vi "MDO-Monitor desktop1.vi"() -> ()   [LabVIEW 2012]
uses:
  SubVI/Controls/main_states.ctl
  SubVI/Controls/Globol_Data_Cluster.ctl
  SubVI/Controls/options.ctl
  SubVI/Controls/main_tab.ctl
  SubVI/Controls/process condition.ctl
  SubVI/Controls/MBA_data.ctl
  <vilib>/Utility/error.llb/DialogType.ctl
  <vilib>/Utility/file.llb/Write To Spreadsheet File (string).vi
  <vilib>/Analysis/baseanly.llb/Mean (DBL).vi
  <vilib>/Analysis/NI_AALBase.lvlib
panel:
  in  "Reset_data":bool
  in  "Пауза":bool
  in  "Принудительный запуск":bool
  in  "Отложенный запуск":bool
  in  "СТОП":bool
  out "ДАННЫЕ СОХРАНЕНЫ":string="ДАННЫЕ СОХРАНЕНЫ"
  in  "Save_data":bool
  in  "ПРИМЕЧАНИЕ":bool
  in  "ТОК ТОЧНО":u8(slide)=5 max=10 step=1 scale=0.0..10.0
  in  "ТОК ГРУБО":u8(slide)=1 max=2 step=1 scale=0.0..2.0
  in  "ПРЕДЕЛЫ ПО НАПРЯЖ":bool=TRUE
  in  "StopUgasanie":bool caption="Остановка по угасанию"
  out "ТАЙМЕР Текущий":string
  out "УГАСАНИЕ":string="УГАСАНИЕ"
  out "ДР":string="Д Р"
  out "ИР":string="И Р"
  out "ГАЛЬВ.ЛЮМ.":string="ГАЛЬВ"
  out "МДР":string="МДР"
  out "СБОР":string="СБОР"
  out "Bounds:Area Width":u32
  in  "СТОП - КАДР":bool
  in  "Graph Tab":T1(tab)
  out "Mixed Signal Graph":T2(graph)
  out "FormCharts":T3(graph) caption="Формовочные кривые"
  out "Process Electrical Parameters":string[][](table)
  out "Bath type":string caption="Ванна"
  out "Electrolyte temperature":dbl(slide) caption="Температура электролита" scale=0.0..60.0
  out "Cooler flow":dbl(knob) caption="Давление воды в системе охлаждения" scale=0.0..3.5 scale format="%#_2g"
  out "Bubbling flow":bool caption="Расход газа в барботере"
  out "Ventilation flow":bool caption="Расход газа в вытяжке"
  out "Application Directory":path
  out "Max_voltage":dbl
  out "states_history":string
  out "current_state":T4
  # "ПАНЕЛЬ ЗАПУСКА"
  # "ПУСК СЛЕДЯЩИЙ"
  # "ПУСК ПРИНУДИТ"
  # "ПАУЗА"
  # "СТОП"
  # "ПАНЕЛЬ ИНДИКАЦИИ"
  # "ПАНЕЛЬ УПРАВЛЕНИЯ"
  # "ПРЕДЕЛЫ\nПО НАПРЯЖ"
  # "800 /200"
  # "1000 / 250"
  # "СОБРАННЕ\nДАННЫЕ"
  # "ПРЕДЕЛЫ\nПО ТОКУ"
  # "ГРУБО"
  # "ТОЧНО"
  # "о"
  # "С"
  # "атм"
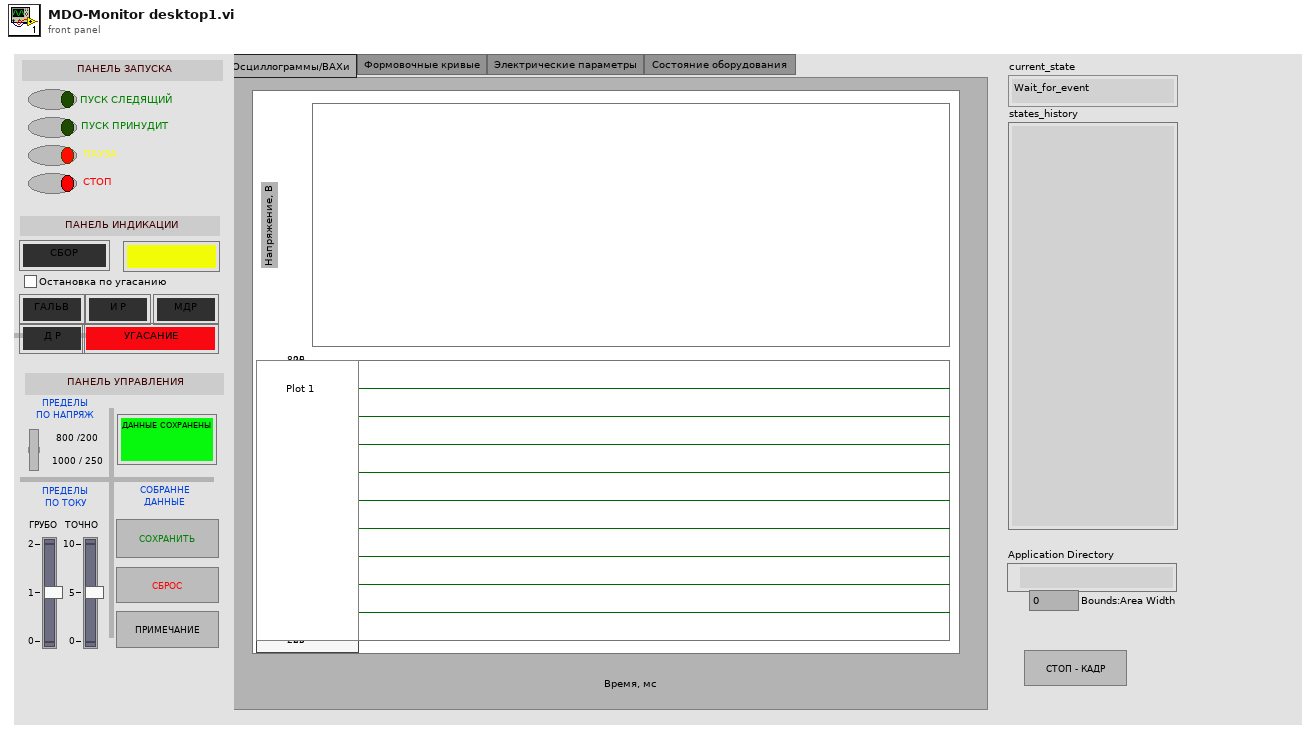
[diagram p1: front panel]
types:
  T1 = enum32{"Осциллограммы/ВАХи", "Формовочные кривые", "Электрические параметры", "Состояние оборудования "}
  T2 = cluster{"Voltege waveform":waveform(dbl), "Current waveform":waveform(dbl)}
  T3 = cluster{"Anod_amp":dbl, "Anod_rms":dbl, "Anod_mean":dbl, "Katod_amp":dbl, "Katod_rms":dbl, "Katod_mean":dbl, "Anod_amp":dbl, "Anod_rms":dbl, "Anod_mean":dbl, "Katod_amp":dbl, "Katod_rms":dbl, "Katod_mean":dbl}
  T4 = typedef "main_states.ctl" = enum16{"Wait_for_event", "Initialize", "Save_ini", "Save_data", "Streaming_config", "Streaming_open", "Streaming_monitor", "Streaming_stop", "Vizualyze", "Form_data_fetch", "Process_analyze", "Start_data_loging", "Pause_data_loging", "Stop_data_loging", "Reset_data_colection", "Error_handler", "Stop", "Settings_dialog"}
  T5 = typedef "Globol_Data_Cluster.ctl" = cluster{"Streaming_enable":bool, "Options":T6, "Ini_file_path":path, "Global_errors":errorcluster, "Main Tab":T7, "Process conditions":T8, "App_directory_path":path, "Data_write_enable":bool, "Process_time":u32, "startup_time":u32, "Streaming Refnum":refnum<vi>, "Note Refnum":refnum<vi>, "Note":string, "Modbus spy Refnum":refnum<vi>, "MBA data":T9, "shutdown?":bool, "Oscil_path":path, " Data log path":path, "Voltege waveform":waveform(dbl), "Current waveform":waveform(dbl)}
  T6 = typedef "options.ctl" = cluster{"Form_data_log_period":i32, "startup_threshold":dbl, "Coeff_U":dbl, "Offset_U":dbl, "Coeff_I":dbl, "Offset_I":dbl, "Save_data_path":path, "ADC_frequency":dbl, "VISA resource name":refnum<visa-resource-name>}
  T7 = typedef "main_tab.ctl" = enum32{"Выбор", "Описание эксперимента", "Монитор", "Визуализатор", "Принтер", "Настройщик"}
  T8 = typedef "process condition.ctl" = cluster{"Data":string, "Time":string, "Subject":string, "Research target":string, "Material":string, "Electrolyte composition":string[][], "MDO mode":string, "Bath volume":string, "Process duration":i32}
  T9 = typedef "MBA_data.ctl" = cluster{"MBA_ch 1":dbl, "MBA_ch 2":dbl, "MBA_ch 3":dbl, "MBA_ch 4":dbl, "MBA_ch 5":dbl, "MBA_ch 6":dbl, "MBA_ch 7":dbl, "MBA_ch 8":dbl}
  T10 = cluster{"Anod_amp":dbl, "Anod_rms":dbl, "Anod_mean":dbl, "Katod_amp":dbl, "Katod_rms":dbl, "Katod_mean":dbl, "Anod_amp":dbl, "Anod_rms":dbl, "Anod_mean":dbl, "Katod_amp":dbl, "Katod_rms":dbl, "Katod_mean":dbl}[]
  T11 = enum16{"open", "replace", "create", "open or create", "replace or create", "replace or create with confirmation"}
  T12 = enum8{"Enabled", "Disabled", "Disabled and Grayed Out"}
  T13 = enum32{"invalid app kind", "Development System", "Run Time System", "Student Edition", "Embedded LabVIEW", "Evaluation", "Custom"}
  T14 = cluster{"Katod_amp":dbl, "Katod_rms":dbl, "Katod_mean":dbl}
  T15 = cluster{"Katod_amp":string, "Katod_rms":string, "Katod_mean":string}
  T16 = cluster{"Anod_amp":dbl, "Anod_rms":dbl, "Anod_mean":dbl}
  T17 = cluster{"Anod_amp":string, "Anod_rms":string, "Anod_mean":string}
  T18 = typedef "DialogType.ctl" = u16
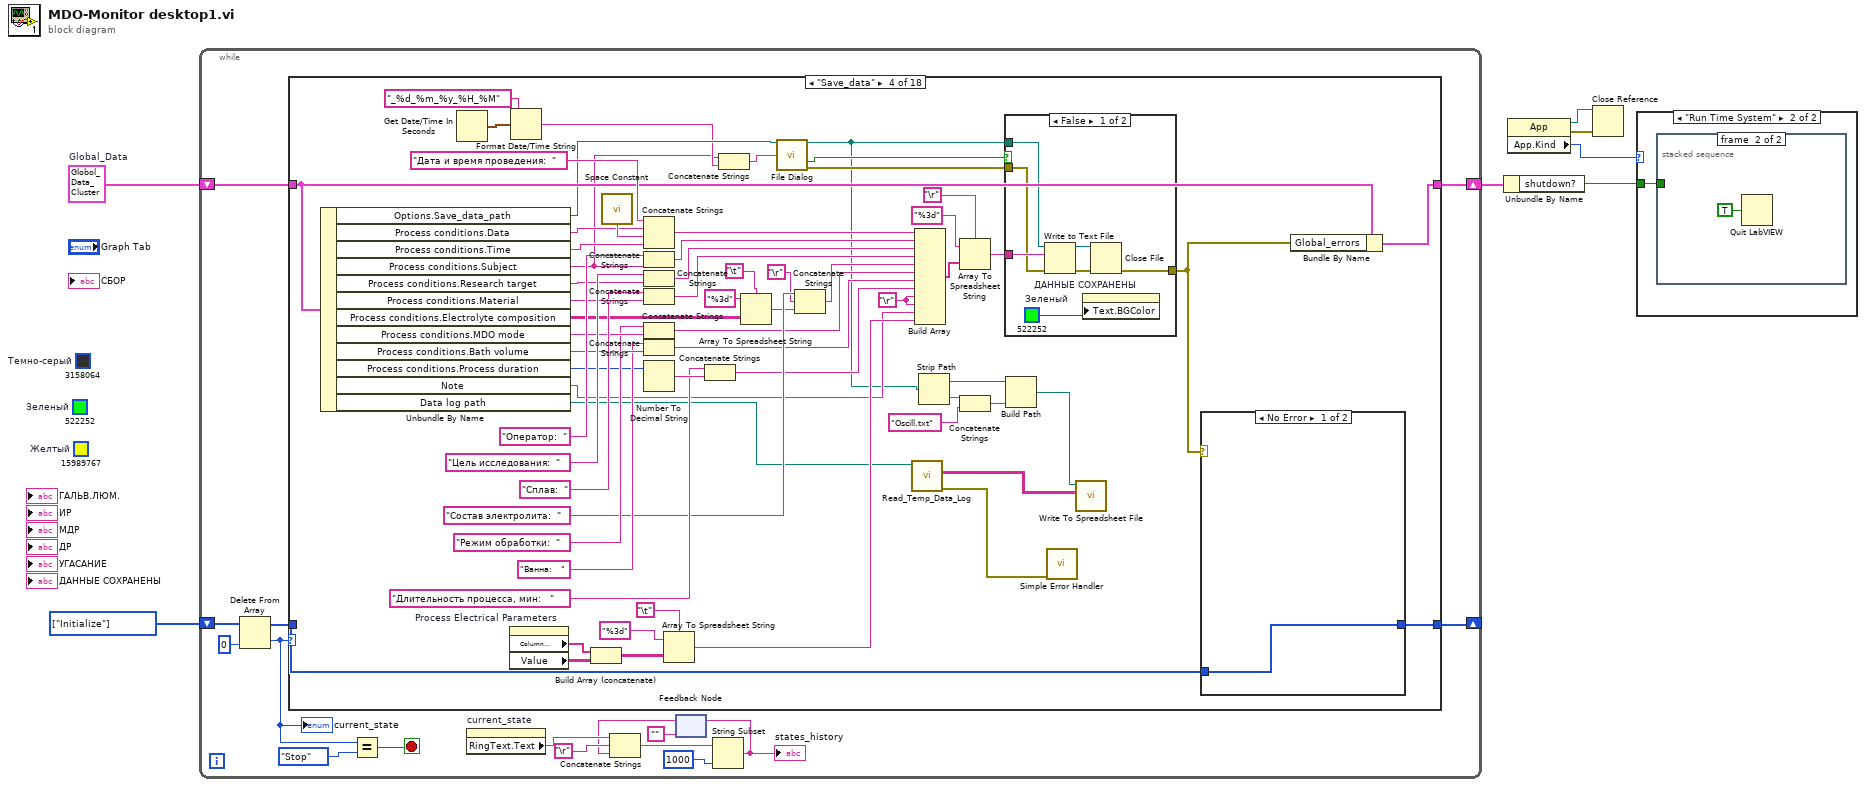
[diagram p0: block diagram]
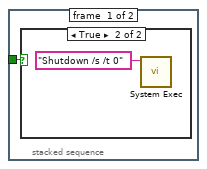
[diagram p3: hidden frame]
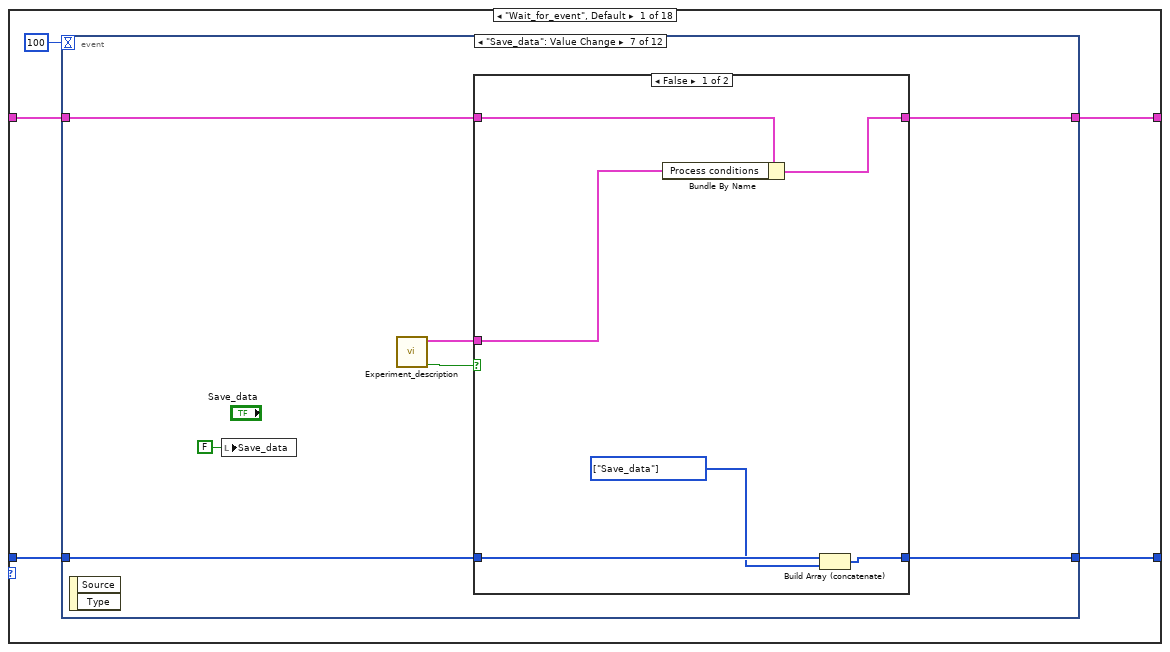
[diagram p5: hidden frame]
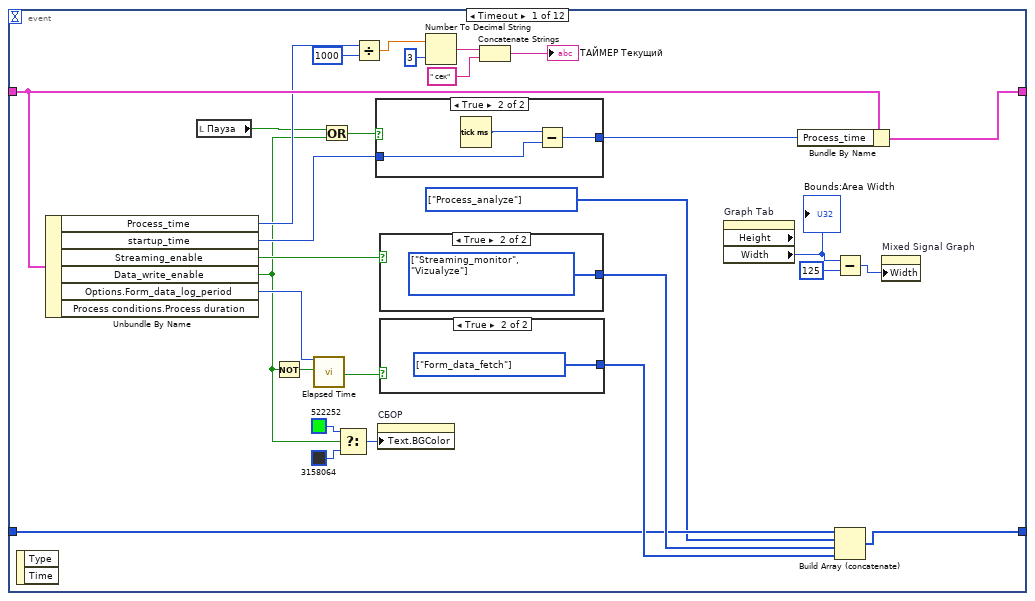
[diagram p6: hidden frame]
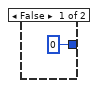
[diagram p7: hidden frame]
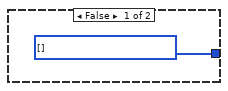
[diagram p8: hidden frame]
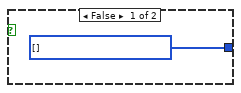
[diagram p9: hidden frame]
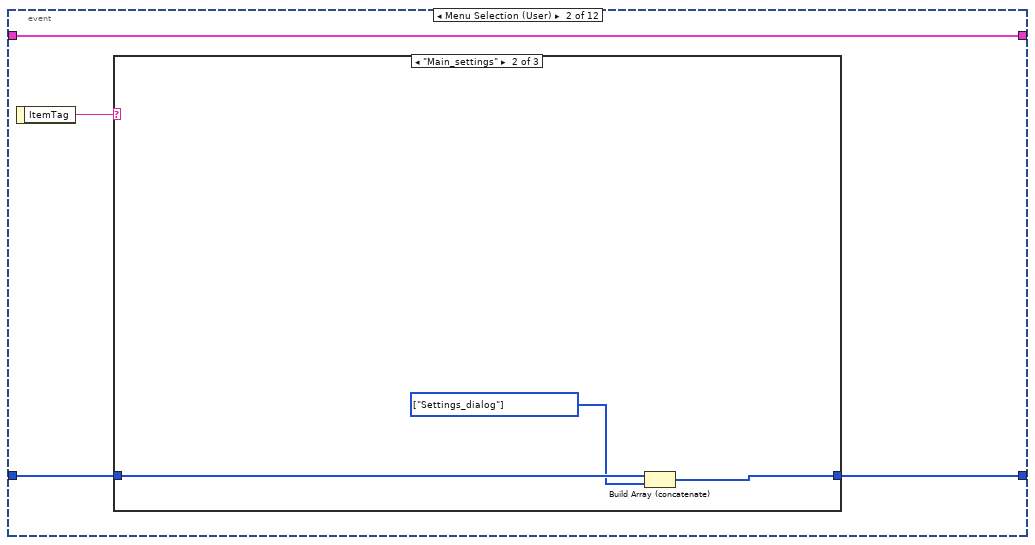
[diagram p10: hidden frame]
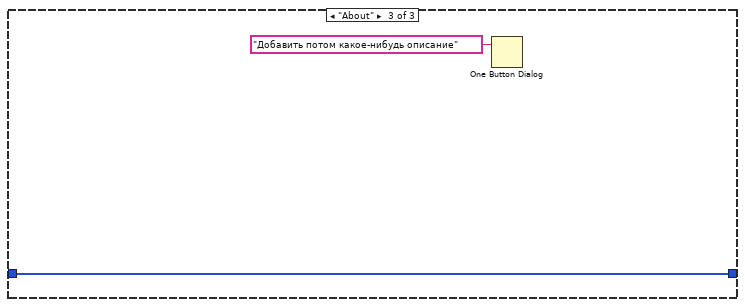
[diagram p12: hidden frame]
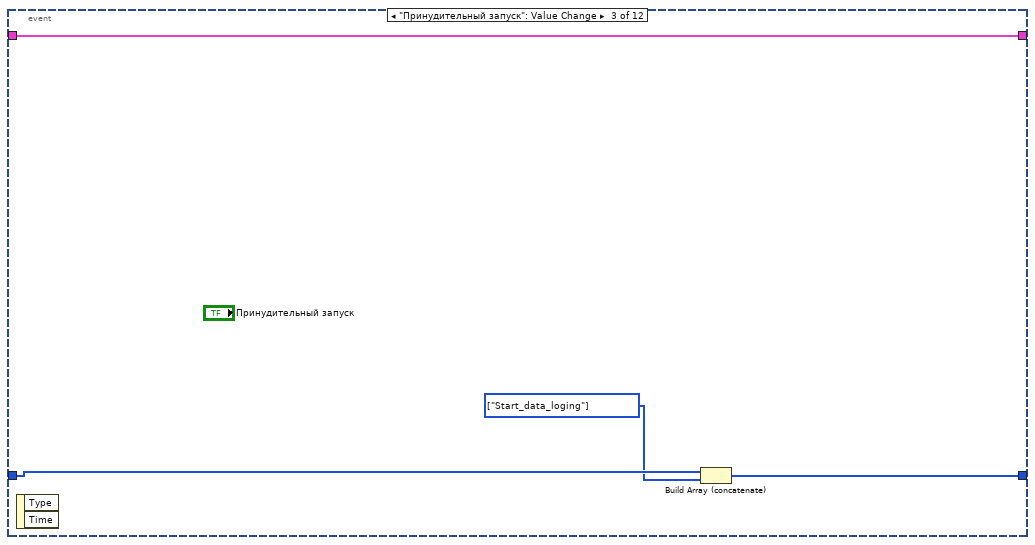
[diagram p13: hidden frame]
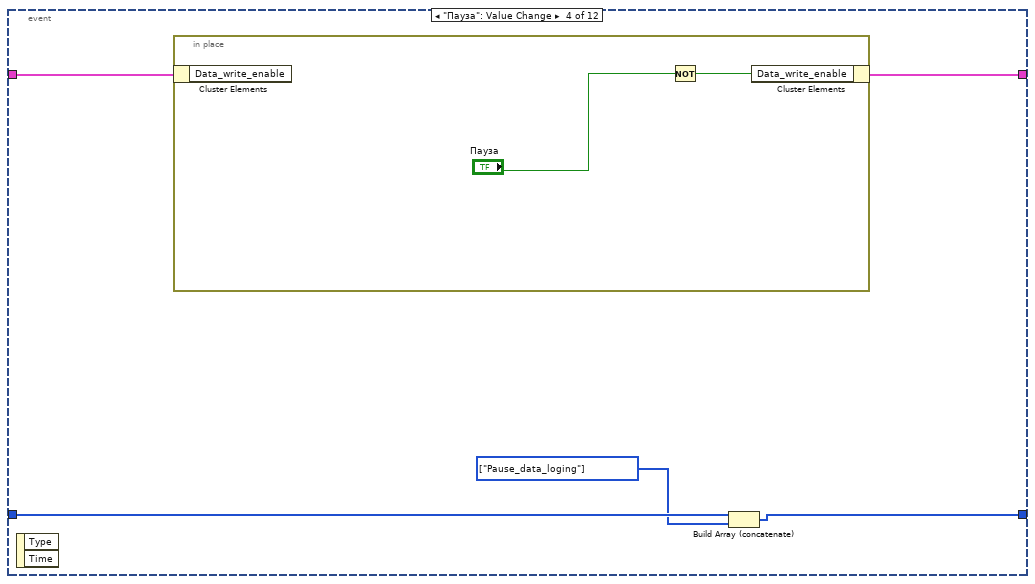
[diagram p14: hidden frame]
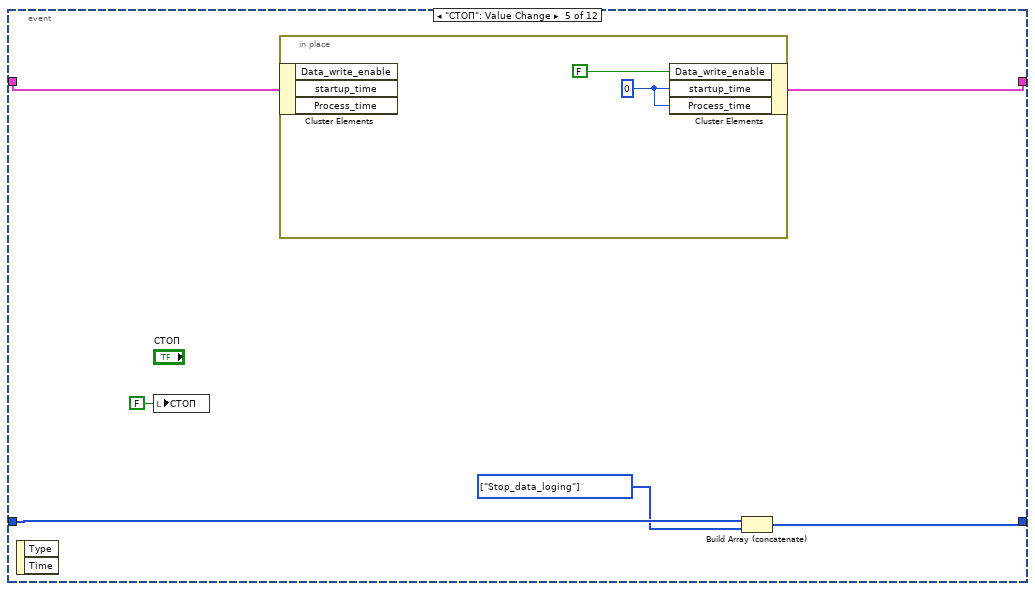
[diagram p15: hidden frame]
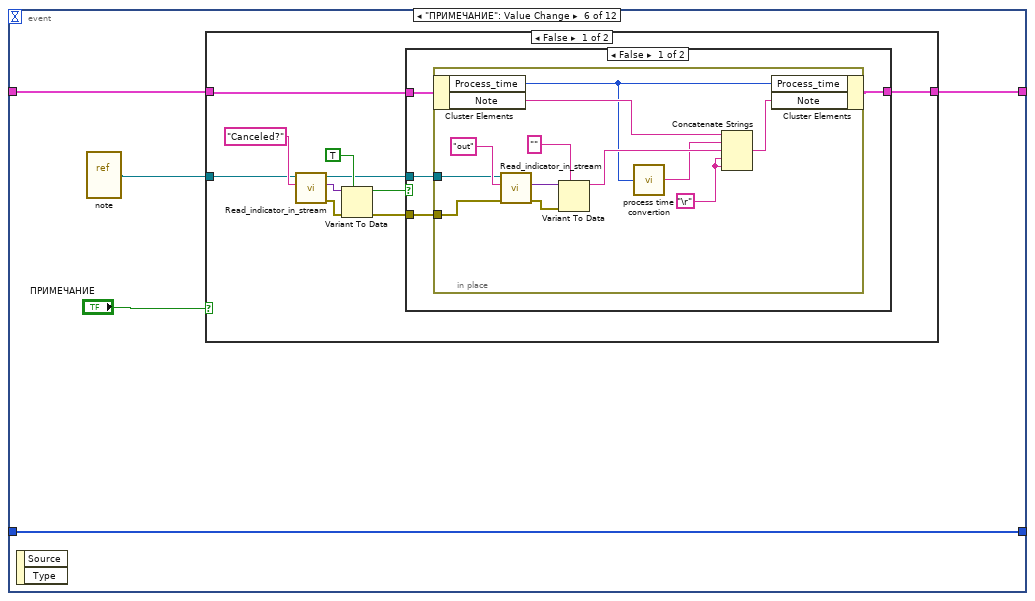
[diagram p16: hidden frame]
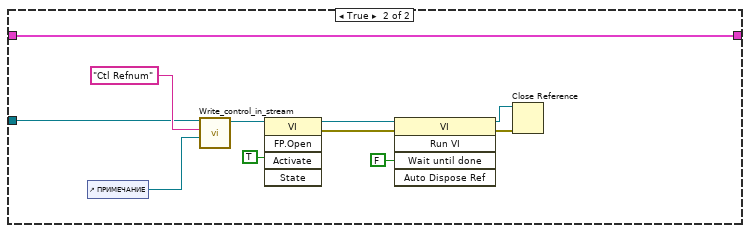
[diagram p18: hidden frame]
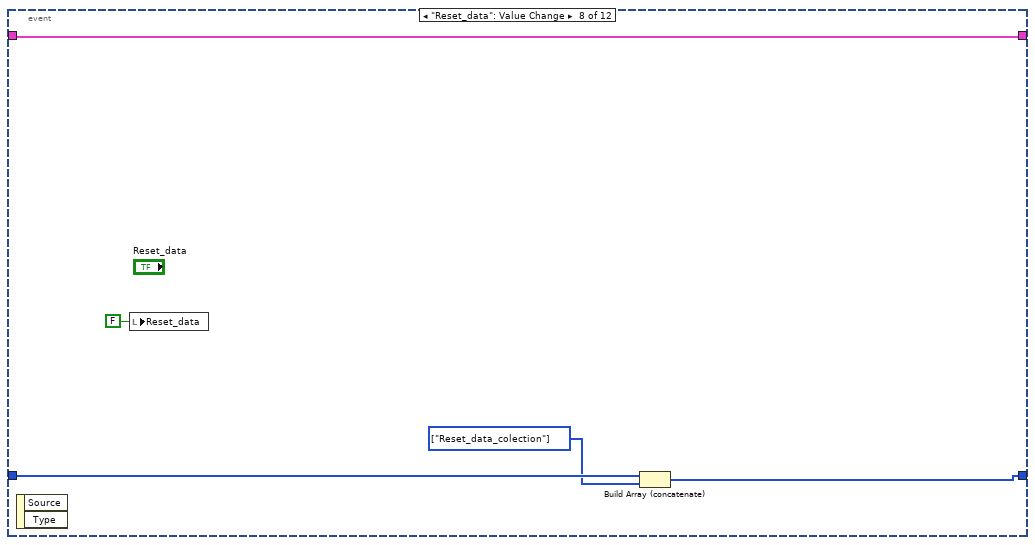
[diagram p20: hidden frame]
diagram:
  (unwired) u32 522252  # Зеленый
  (unwired) u32 15989767  # Желтый
  (unwired) u32 3158064  # Темно-серый
  w6 = T5 {"Streaming_enable"=FALSE, "Options"={"Form_data_log_period"=0, "startup_threshold"=0.0, "Coeff_U"=0.0, "Offset_U"=0.0, "Coeff_I"=0.0, "Offset_I"=0.0, "Save_data_path"=path "", "ADC_frequency"=0.0, "VISA resource name"=""}, "Ini_file_path"=path "", "Global_errors"={"status"=FALSE, "code"=0, "source"=""}, "Main Tab"=enum."Выбор", "Process conditions"={"Data"="", "Time"="", "Subject"="", "Research target"="", "Material"="", "Electrolyte composition"=[], "MDO mode"="", "Bath volume"="", "Process duration"=0}, "App_directory_path"=path "", "Data_write_enable"=FALSE, "Process_time"=0, "startup_time"=0, "Streaming Refnum"=refnum, "Note Refnum"=refnum, "Note"="", "Modbus spy Refnum"=refnum, "MBA data"={"MBA_ch 1"=0.0, "MBA_ch 2"=0.0, "MBA_ch 3"=0.0, "MBA_ch 4"=0.0, "MBA_ch 5"=0.0, "MBA_ch 6"=0.0, "MBA_ch 7"=0.0, "MBA_ch 8"=0.0}, "shutdown?"=FALSE, "Oscil_path"=path "", " Data log path"=path "", "Voltege waveform"={"t0"=timestamp(0 s since 1904-01-01), "dt"=1.0, "Y"=[]}, "Current waveform"={"t0"=timestamp(0 s since 1904-01-01), "dt"=1.0, "Y"=[]}}  # Global_Data
  w7 = T4[] [enum."Initialize"] items=["Wait_for_event", "Initialize", "Save_ini", "Save_data", "Streaming_config", "Streaming_open", "Streaming_monitor", "Streaming_stop", "Vizualyze", "Form_data_fetch", "Process_analyze", "Start_data_loging", "Pause_data_loging", "Stop_data_loging", "Reset_data_colection", "Error_handler", "Stop", "Settings_dialog"]
  n1 = while {
    shift-right: [w15] -> w5
    shift-left: w6 -> [w16]
    shift-right: [w9] -> _
    shift-left: w7 -> [w10]
    stop <- w23 stop-if-true
    n2 = Delete From Array(array=w10, index=0) -> (deleted portion=w8:T4, array with subset deleted=w14:T4[])  [unwired: 1 in]
    "current_state" <- w8
    n3 = case shown="\"Save_data\"" w8 {
      tunnel: w16 -> [w27 w223 w240 w273 w331 w361 w403 w433 w467 w514 w550 w603 w611 w614 w619 w630 w641 w647]
      tunnel: [w26 w219 w238 w272 w330 w363 w404 w435 w467 w514 w550 w602 w611 w614 w619 w629 w641 w643] -> w15
      tunnel: w14 -> [w25 w222 w236 w271 w333 w364 w406 w430 w460 w529 w549 w604 w612 w615 w626 w628 w642 w646]
      tunnel: [w24 w221 w235 w270 w332 w364 w405 w429 w459 w529 w548 w604 w612 w615 w626 w627 w642 w644] -> w9
      frame "Wait_for_event", Default {
        n4 = event shown="[6] \"Save_data\": Value Change" {
          selector: _ -> [_ _ _ _ _ _ _ _ _ _ _ _]
          dyn-events: _ -> [_ _ _ _ _ _ _ _ _ _ _ _]
          timeout: 100 -> [_ _ _ _ _ _ _ _ _ _ _ _]
          tunnel: w27 -> [w50 w69 w79 w81 w89 w98 w141 w156 w160 w168 w183 w187]
          tunnel: [w49 w69 w79 w80 w88 w97 w140 w156 w160 w168 w183 w187] -> w26
          tunnel: w25 -> [w42 w67 w78 w84 w92 w99 w144 w155 w161 w167 w182 w185]
          tunnel: [w51 w66 w76 w82 w91 w99 w143 w154 w161 w167 w182 w184] -> w24
          event Timeout {
            w41 = T4[] [enum."Process_analyze"] items=["Wait_for_event", "Initialize", "Save_ini", "Save_data", "Streaming_config", "Streaming_open", "Streaming_monitor", "Streaming_stop", "Vizualyze", "Form_data_fetch", "Process_analyze", "Start_data_loging", "Pause_data_loging", "Stop_data_loging", "Reset_data_colection", "Error_handler", "Stop", "Settings_dialog"] ("array")
            n5 = event-data() -> ()  [unwired: 1 in, 2 out]
            n6 = Unbundle By Name(w50) -> ("Process_time"=w40:u32, "startup_time"=w36:u32, "Streaming_enable"=w57:bool, "Data_write_enable"=w34:bool, "Options.Form_data_log_period"=w55:i32)  [unwired: 1 out]
            n7 = local read "Пауза"() -> (w32:bool)
            n8 = Not(x=w34) -> (.not. x?=w56:bool)
            n9 = call "Elapsed Time"("Time Target (s)"=w55, "Reset"=w56) -> ("Time has Elapsed"=w54:bool)  [unwired: 10 in, 7 out]
            n10 = Or(x=w32, y=w34) -> (x .or. y?=w33:bool)
            n11 = Select(t=u32 522252 ("Зеленый"), s=w34, f=u32 3158064) -> (s? t:f=w37:u32)
            n12 = Divide(x=w40, y=u32 1000) -> (x/y=w44:dbl)
            n13 = case shown="True" w33 {
              tunnel: w36 -> [_ w60]
              tunnel: [u32 0 w59] -> w35
              frame False {
              }
              frame True {
                n14 = Tick Count (ms)() -> (millisecond timer value=w61:u32)
                n15 = Subtract(x=w61, y=w60) -> (x-y=w59:u32)
              }
            }
            n16 = property on="СБОР" class="Str"("Text.BGColor"=w37) -> ()  [unwired: 2 in, 2 out]
            n17 = case shown="True" w57 {
              tunnel: [w64 w65] -> w53
              frame False {
                w64 = T4[] [] items=["Wait_for_event", "Initialize", "Save_ini", "Save_data", "Streaming_config", "Streaming_open", "Streaming_monitor", "Streaming_stop", "Vizualyze", "Form_data_fetch", "Process_analyze", "Start_data_loging", "Pause_data_loging", "Stop_data_loging", "Reset_data_colection", "Error_handler", "Stop", "Settings_dialog"] ("array")
              }
              frame True {
                w65 = T4[] [enum."Streaming_monitor", enum."Vizualyze"] items=["Wait_for_event", "Initialize", "Save_ini", "Save_data", "Streaming_config", "Streaming_open", "Streaming_monitor", "Streaming_stop", "Vizualyze", "Form_data_fetch", "Process_analyze", "Start_data_loging", "Pause_data_loging", "Stop_data_loging", "Reset_data_colection", "Error_handler", "Stop", "Settings_dialog"] ("array")
              }
            }
            n18 = case shown="True" w54 {
              tunnel: [w62 w63] -> w52
              frame False {
                w62 = T4[] [] items=["Wait_for_event", "Initialize", "Save_ini", "Save_data", "Streaming_config", "Streaming_open", "Streaming_monitor", "Streaming_stop", "Vizualyze", "Form_data_fetch", "Process_analyze", "Start_data_loging", "Pause_data_loging", "Stop_data_loging", "Reset_data_colection", "Error_handler", "Stop", "Settings_dialog"] ("array")
              }
              frame True {
                w63 = T4[] [enum."Form_data_fetch"] items=["Wait_for_event", "Initialize", "Save_ini", "Save_data", "Streaming_config", "Streaming_open", "Streaming_monitor", "Streaming_stop", "Vizualyze", "Form_data_fetch", "Process_analyze", "Start_data_loging", "Pause_data_loging", "Stop_data_loging", "Reset_data_colection", "Error_handler", "Stop", "Settings_dialog"] ("array")
              }
            }
            n19 = Number To Decimal String(number=w44, width (-)=i16 3) -> (decimal integer string=w46:string)
            n20 = Concatenate Strings(w46, " сек" ("string")) -> (→"ТАЙМЕР Текущий":string)
            n21 = property on="Graph Tab" class="TabCtl (strict)" props=["Height", "Width"]() -> ("Width"=w31:u32)  [unwired: 2 in, 3 out]
            "Bounds:Area Width" <- w31
            n22 = Bundle By Name(cluster=w50, "Process_time"=w35) -> (w49:T5)
            n23 = Subtract(x=w31, y=u32 125) -> (x-y=w30:u32)
            n24 = Build Array (concatenate)(w42, w41, w53, w52) -> (w51:T4[])
            n25 = property on="Mixed Signal Graph" class="MixedGraph (strict)"("Width"=w30) -> ()  [unwired: 2 in, 2 out]
          }
          event Menu Selection (User) {
            n26 = event-data() -> ("ItemTag"=w68:string)  [unwired: 1 in]
            n27 = case shown="\"Main_settings\"" w68 {
              tunnel: w67 -> [w70 w73 w74]
              tunnel: [w70 w71 w74] -> w66
              frame Default {
              }
              frame "Main_settings" {
                w72 = T4[] [enum."Settings_dialog"] items=["Wait_for_event", "Initialize", "Save_ini", "Save_data", "Streaming_config", "Streaming_open", "Streaming_monitor", "Streaming_stop", "Vizualyze", "Form_data_fetch", "Process_analyze", "Start_data_loging", "Pause_data_loging", "Stop_data_loging", "Reset_data_colection", "Error_handler", "Stop", "Settings_dialog"] ("array")
                n28 = Build Array (concatenate)(w73, w72) -> (w71:T4[])
              }
              frame "About" {
                n29 = One Button Dialog(message="Добавить потом какое-нибудь описание") -> ()  [unwired: 1 in, 1 out]
              }
            }
          }
          event "Принудительный запуск": Value Change {
            w77 = T4[] [enum."Start_data_loging"] items=["Wait_for_event", "Initialize", "Save_ini", "Save_data", "Streaming_config", "Streaming_open", "Streaming_monitor", "Streaming_stop", "Vizualyze", "Form_data_fetch", "Process_analyze", "Start_data_loging", "Pause_data_loging", "Stop_data_loging", "Reset_data_colection", "Error_handler", "Stop", "Settings_dialog"] ("array")
            n30 = event-data() -> ()  [unwired: 1 in, 2 out]
            n31 = Build Array (concatenate)(w78, w77) -> (w76:T4[])
          }
          event "Пауза": Value Change {
            w83 = T4[] [enum."Pause_data_loging"] items=["Wait_for_event", "Initialize", "Save_ini", "Save_data", "Streaming_config", "Streaming_open", "Streaming_monitor", "Streaming_stop", "Vizualyze", "Form_data_fetch", "Process_analyze", "Start_data_loging", "Pause_data_loging", "Stop_data_loging", "Reset_data_colection", "Error_handler", "Stop", "Settings_dialog"] ("array")
            n32 = event-data() -> ()  [unwired: 1 in, 2 out]
            n33 = in-place {
              n34 = in-place-cluster #1(w81) -> ()  [unwired: 1 out]
              n35 = Not(x="Пауза") -> (.not. x?=w85:bool)
              n36 = in-place-cluster #1("Data_write_enable"=w85) -> (w80:T5)
            }
            n37 = Build Array (concatenate)(w84, w83) -> (w82:T4[])
          }
          event "СТОП": Value Change {
            w90 = T4[] [enum."Stop_data_loging"] items=["Wait_for_event", "Initialize", "Save_ini", "Save_data", "Streaming_config", "Streaming_open", "Streaming_monitor", "Streaming_stop", "Vizualyze", "Form_data_fetch", "Process_analyze", "Start_data_loging", "Pause_data_loging", "Stop_data_loging", "Reset_data_colection", "Error_handler", "Stop", "Settings_dialog"] ("array")
            n38 = event-data() -> ()  [unwired: 1 in, 2 out]
            n39 = local write "СТОП"(FALSE ("СТОП")) -> ()
            n40 = in-place {
              w93 = u32 0 ("startup_time")
              n41 = in-place-cluster #2(w89) -> ()  [unwired: 3 out]
              n42 = in-place-cluster #2("Data_write_enable"=FALSE, "startup_time"=w93, "Process_time"=w93) -> (w88:T5)
            }
            n43 = Build Array (concatenate)(w92, w90) -> (w91:T4[])
          }
          event "ПРИМЕЧАНИЕ": Value Change {
            n44 = event-data() -> ()  [unwired: 1 in, 2 out]
            n45 = vi-ref "note.vi"() -> (w95:refnum<vi>)
            n46 = case shown="False" "ПРИМЕЧАНИЕ" {
              tunnel: w98 -> [w109 w135]
              tunnel: [w108 w135] -> w97
              tunnel: w95 -> [w104 w127]
              frame False {
                n47 = call "Read_indicator_in_stream.vi"("Required_indicatorl_name"="Canceled?", "reference"=w104) -> ("error out"=w101:errorcluster, "Value"=w106:variant, "reference out"=w102:refnum<vi>)  [unwired: 7 in]
                n48 = Variant To Data(error in=w101, type=TRUE, Variant=w106) -> (data=w103:bool, error out=w100:errorcluster)
                n49 = case shown="False" w103 {
                  tunnel: w109 -> [w113 w126]
                  tunnel: [w112 w126] -> w108
                  tunnel: w102 -> [w111 _]
                  tunnel: w100 -> [w110 _]
                  frame False {
                    n50 = in-place {
                      in-place-border: w111 -> [w117]
                      in-place-border: w110 -> [w116]
                      w124 = "\r"
                      n51 = in-place-cluster #3(w113) -> ("Process_time"=w115:u32, "Note"=w118:string)
                      n52 = call "Read_indicator_in_stream.vi"("error in (no error)"=w116, "Required_indicatorl_name"="out", "reference"=w117) -> ("error out"=w121:errorcluster, "Value"=w122:variant)  [unwired: 6 in, 1 out]
                      n53 = Variant To Data(error in=w121, type="" ("string"), Variant=w122) -> (data=w120:string)  [unwired: 1 out]
                      n54 = call "process time convertion.vi"("process_time"=w115) -> ("out"=w114:string)
                      n55 = Concatenate Strings(w118, w114, w120, w124, w124) -> (w125:string)
                      n56 = in-place-cluster #3("Process_time"=w115, "Note"=w125) -> (w112:T5)
                    }
                  }
                  frame True {
                  }
                }
              }
              frame True {
                n57 = control-ref of="ПРИМЕЧАНИЕ"() -> (w128:refnum<vi>)
                n58 = call "Write_control_in_stream.vi"("Value"=w128, "Required_control_name"="Ctl Refnum", "reference"=w127) -> ("reference out"=w130:refnum<vi>)  [unwired: 8 in]
                n59 = invoke class="VI" method="FP.Open"(reference=w130, "Activate"=TRUE ("Activate?")) -> (reference out=w133:refnum<vi>, error out=w131:errorcluster)  [unwired: 3 in, 3 out]
                n60 = invoke class="VI" method="Run VI"(reference=w133, error in=w131, "Wait until done"=FALSE ("Wait Until Done")) -> (reference out=w134:refnum<vi>, error out=w137:errorcluster)  [unwired: 2 in, 3 out]
                n61 = Close Reference(reference=w134, error in (no error)=w137) -> ()  [unwired: 1 out]
              }
            }
          }
          event "Save_data": Value Change {
            n62 = event-data() -> ()  [unwired: 1 in, 2 out]
            n63 = local write "Save_data"(FALSE ("Save_data")) -> ()
            n64 = call "Experiment_description.vi"() -> ("Canceled"=w139:bool, "Process conditions"=w138:T8)  [unwired: 10 in]
            n65 = case shown="False" w139 {
              tunnel: w144 -> [w150 w151]
              tunnel: [w149 w151] -> w143
              tunnel: w141 -> [w147 w152]
              tunnel: [w145 w152] -> w140
              tunnel: w138 -> [w146 _]
              frame False {
                w148 = T4[] [enum."Save_data"] items=["Wait_for_event", "Initialize", "Save_ini", "Save_data", "Streaming_config", "Streaming_open", "Streaming_monitor", "Streaming_stop", "Vizualyze", "Form_data_fetch", "Process_analyze", "Start_data_loging", "Pause_data_loging", "Stop_data_loging", "Reset_data_colection", "Error_handler", "Stop", "Settings_dialog"] ("array")
                n66 = Bundle By Name(cluster=w147, "Process conditions"=w146) -> (w145:T5)
                n67 = Build Array (concatenate)(w150, w148) -> (w149:T4[])
              }
              frame True {
              }
            }
          }
          event "Reset_data": Value Change {
            w153 = T4[] [enum."Reset_data_colection"] items=["Wait_for_event", "Initialize", "Save_ini", "Save_data", "Streaming_config", "Streaming_open", "Streaming_monitor", "Streaming_stop", "Vizualyze", "Form_data_fetch", "Process_analyze", "Start_data_loging", "Pause_data_loging", "Stop_data_loging", "Reset_data_colection", "Error_handler", "Stop", "Settings_dialog"] ("array")
            n68 = event-data() -> ()  [unwired: 1 in, 2 out]
            n69 = local write "Reset_data"(FALSE ("Reset_data")) -> ()
            n70 = Build Array (concatenate)(w155, w153) -> (w154:T4[])
          }
          event "СТОП - КАДР": Value Change {
            n71 = event-data() -> ()  [unwired: 1 in, 2 out]
            n72 = local write "СТОП - КАДР"(FALSE ("СТОП - КАДР")) -> ()
            n73 = One Button Dialog(message="Эта функция пока не работает") -> ()  [unwired: 1 in, 1 out]
          }
          event "ПРЕДЕЛЫ ПО НАПРЯЖ": Value Change {
            n74 = event-data() -> ()  [unwired: 1 in, 2 out]
            n75 = case shown="False" "ПРЕДЕЛЫ ПО НАПРЯЖ" {
              tunnel: [999.0 ("Y Scale.Range:Maximum") 800.0 ("Y Scale.Range:Maximum")] -> w162
              tunnel: [-250.0 ("Y Scale.Range:Minimum") -200.0 ("Y Scale.Range:Minimum")] -> w164
              frame False {
              }
              frame True {
              }
            }
            n76 = property on="Mixed Signal Graph" class="MixedGraph (strict)"("ActYScl"=0 ("Active Y Scale"), "YScale.Maximum"=w162, "YScale.Minimum"=w164) -> ()  [unwired: 2 in, 2 out]
            n77 = property on="FormCharts" class="WFChart (strict)"("ActYScl"=0 ("Active Y Scale"), "YScale.Maximum"=w162) -> ()  [unwired: 2 in, 2 out]
          }
          event "ТОК ГРУБО", "ТОК ТОЧНО": Value Change {
            n78 = event-data() -> ()  [unwired: 1 in, 2 out]
            n79 = Increment(x="ТОК ГРУБО") -> (x+1=w177:u8)
            n80 = Multiply(x=10.0, y=w177) -> (x*y=w180:dbl)
            n81 = Add(x=w180, y="ТОК ТОЧНО") -> (x+y=w173:dbl)
            n82 = Negate(x=w173) -> (-x=w175:dbl)
            n83 = property on="FormCharts" class="WFChart (strict)"("ActYScl"=1 ("Active Y Scale"), "YScale.Maximum"=w173) -> ()  [unwired: 2 in, 2 out]
            n84 = property on="Mixed Signal Graph" class="MixedGraph (strict)"("ActYScl"=1 ("Active Y Scale"), "YScale.Maximum"=w173, "YScale.Minimum"=w175) -> ()  [unwired: 2 in, 2 out]
          }
          event Panel Close? {
            n85 = event-data() -> ()  [unwired: 1 in, 2 out]
            n86 = Two Button Dialog(message="Вы действительно хотите закрыть программу?", 1:"Нет" ("F button name (\"Cancel\")"), 2:"Да" ("T button name (\"OK\")")) -> (T button?=w186:bool)
            n87 = case shown="True" w186 {
              tunnel: w185 -> [w192 w195]
              tunnel: [w192 w194] -> w184
              frame False {
              }
              frame True {
                w193 = T4[] [enum."Streaming_stop", enum."Stop"] items=["Wait_for_event", "Initialize", "Save_ini", "Save_data", "Streaming_config", "Streaming_open", "Streaming_monitor", "Streaming_stop", "Vizualyze", "Form_data_fetch", "Process_analyze", "Start_data_loging", "Pause_data_loging", "Stop_data_loging", "Reset_data_colection", "Error_handler", "Stop", "Settings_dialog"] ("array")
                n88 = Build Array (concatenate)(w195, w193) -> (w194:T4[])
              }
            }
            n89 = event-data("Discard?"=TRUE) -> ()  [unwired: 1 in, 1 out]
          }
        }
      }
      frame "Initialize" {
        w197 = T12."Disabled" ("Disabled")
        w215 = u32 3158064 ("Темно-серый")
        w214 = FALSE ("Streaming_enable")
        n90 = property class="App"() -> (reference out=w216:refnum<vi>, error out=w217:errorcluster, "App.Kind"=w224:T13)  [unwired: 2 in]
        n91 = Close Reference(reference=w216, error in (no error)=w217) -> ()  [unwired: 1 out]
        n92 = case shown="\"Development System\", Default" w224 {
          tunnel: [w231 w233] -> w201
          frame "Development System", Default {
            n93 = Current VI's Path() -> (path=w232:path)
            n94 = Strip Path(path=w232) -> (stripped path=w231:path)  [unwired: 1 out]
          }
          frame "Run Time System" {
            n95 = call <vilib>:"Application Directory.vi"() -> ("Application Directory"=w233:path)
          }
        }
        "Application Directory" <- w201
        n96 = property on="Mixed Signal Graph" class="MixedGraph (strict)"("ScaleLegendVis"=FALSE ("Scale Legend:Visible")) -> ()  [unwired: 2 in, 2 out]
        n97 = property on="Пауза" class="Bool (strict)"("DisabledEnum"=w197) -> ()  [unwired: 2 in, 2 out]
        n98 = property on="СТОП" class="Bool (strict)"("DisabledEnum"=w197) -> ()  [unwired: 2 in, 2 out]
        n99 = property on="FormCharts" class="WFChart (strict)"("History Data"=T10 []) -> ()  [unwired: 2 in, 2 out]
        n100 = invoke on="Process Electrical Parameters" class="Tbl (strict)" method="Reinit To Default"() -> ()  [unwired: 3 in, 3 out]
        n101 = Build Path(base path=w201, name or relative path="TempDataLog.dat") -> (appended path=w209:path)
        n102 = property on="СБОР" class="Str"("Text.BGColor"=w215) -> ()  [unwired: 2 in, 2 out]
        n103 = property on="МДР" class="Str"("Text.BGColor"=w215) -> ()  [unwired: 2 in, 2 out]
        n104 = property on="ДР" class="Str"("Text.BGColor"=w215) -> ()  [unwired: 2 in, 2 out]
        n105 = property on="УГАСАНИЕ" class="Str"("Text.BGColor"=w215) -> ()  [unwired: 2 in, 2 out]
        n106 = property on="ГАЛЬВ.ЛЮМ." class="Str"("Text.BGColor"=w215) -> ()  [unwired: 2 in, 2 out]
        n107 = property on="ИР" class="Str"("Text.BGColor"=w215) -> ()  [unwired: 2 in, 2 out]
        n108 = property on="ДАННЫЕ СОХРАНЕНЫ" class="Str"("Text.BGColor"=w215) -> ()  [unwired: 2 in, 2 out]
        n109 = Open/Create/Replace Datalog(5:cluster{string, "empty array":sgl[]} {"", "empty array"=[]}, 10:T11."replace or create" ("operation (0:open)"), 11:w209) -> (0:w207:errorcluster, 3:w206:refnum<k1>)  [unwired: 1 in, 3 out]
        n110 = Build Path(base path=w201, name or relative path="MDO-Toolkit_startup.ini") -> (appended path=w199:path)
        n111 = vi-ref "streaming_demo.vi"() -> (w203:refnum<vi>)
        n112 = vi-ref "streaming_x502.vi"() -> ()  [unwired: 1 out]
        n113 = vi-ref "Modbus_spy.vi"() -> ()  [unwired: 1 out]
        n114 = vi-ref "Modbus_spy_new.vi"() -> (w212:refnum<vi>)
        n115 = Close File(refnum=w206, error in=w207) -> (path=w205:path, error out=w204:errorcluster)
        n116 = call "Read_INI.vi"("error in (no error)"=w204, "App_directory"=w199) -> ("error out"=w220:errorcluster, "Options"=w213:T6, "file path"=w218:path)  [unwired: 7 in]
        n117 = case shown="No Error" w220 {
          tunnel: w222 -> [w227 w229]
          tunnel: [w226 w230] -> w221
          frame No Error {
            w225 = T4[] [enum."Streaming_config", enum."Streaming_open"] items=["Wait_for_event", "Initialize", "Save_ini", "Save_data", "Streaming_config", "Streaming_open", "Streaming_monitor", "Streaming_stop", "Vizualyze", "Form_data_fetch", "Process_analyze", "Start_data_loging", "Pause_data_loging", "Stop_data_loging", "Reset_data_colection", "Error_handler", "Stop", "Settings_dialog"] ("array")
            n118 = Build Array (concatenate)(w227, w225) -> (w226:T4[])
          }
          frame Error {
            w228 = T4[] [enum."Error_handler"] items=["Wait_for_event", "Initialize", "Save_ini", "Save_data", "Streaming_config", "Streaming_open", "Streaming_monitor", "Streaming_stop", "Vizualyze", "Form_data_fetch", "Process_analyze", "Start_data_loging", "Pause_data_loging", "Stop_data_loging", "Reset_data_colection", "Error_handler", "Stop", "Settings_dialog"] ("array")
            n119 = Build Array (concatenate)(w228, w229) -> (w230:T4[])
          }
        }
        n120 = Bundle By Name(cluster=w223, "App_directory_path"=w201, "Data_write_enable"=w214, "Streaming_enable"=w214, "Options"=w213, "Ini_file_path"=w218, "Global_errors"=w220, "Streaming Refnum"=w203, "Modbus spy Refnum"=w212, "Data log path"=w205, "Process_time"=u32 0) -> (w219:T5)
      }
      frame "Save_ini" {
        n121 = Unbundle By Name(w240) -> ("Ini_file_path"=w241:path, "Options"=w234:T6)
        n122 = call "Write_INI.vi"("Options"=w234, "Ini_file_path"=w241) -> ("error out"=w237:errorcluster, "Ini_file_path_out"=w239:path)  [unwired: 8 in]
        n123 = case shown="No Error" w237 {
          tunnel: w236 -> [w242 w243]
          tunnel: [w242 w245] -> w235
          frame No Error {
          }
          frame Error {
            w244 = T4[] [enum."Error_handler"] items=["Wait_for_event", "Initialize", "Save_ini", "Save_data", "Streaming_config", "Streaming_open", "Streaming_monitor", "Streaming_stop", "Vizualyze", "Form_data_fetch", "Process_analyze", "Start_data_loging", "Pause_data_loging", "Stop_data_loging", "Reset_data_colection", "Error_handler", "Stop", "Settings_dialog"] ("array")
            n124 = Build Array (concatenate)(w244, w243) -> (w245:T4[])
          }
        }
        n125 = Bundle By Name(cluster=w240, "Ini_file_path"=w239, "Global_errors"=w237) -> (w238:T5)
      }
      frame "Save_data" {
        w276 = "\r"
        n126 = Unbundle By Name(w273) -> ("Options.Save_data_path"=w267:path, "Process conditions.Data"=w252:string, "Process conditions.Time"=w251:string, "Process conditions.Subject"=w247:string, "Process conditions.Research target"=w253:string, "Process conditions.Material"=w307:string, "Process conditions.Electrolyte composition"=w298:string[][], "Process conditions.MDO mode"=w305:string, "Process conditions.Bath volume"=w303:string, "Process conditions.Process duration"=w301:i32, "Note"=w268:string, "Data log path"=w257:path)
        n127 = Get Date/Time In Seconds() -> (seconds since 1Jan1904=w250:timestamp)
        n128 = property on="Process Electrical Parameters" class="Tbl (strict)"() -> ("Column Headers[]"=w278:string[], "Value"=w279:string[][])  [unwired: 2 in, 2 out]
        n129 = Format Date/Time String(time format string (%c)="_%d_%m_%y_%H_%M", seconds (now)=w250) -> (date/time string=w248:string)  [unwired: 1 in]
        n130 = Build Array (concatenate)(w278, w279) -> (w277:string[][])
        n131 = call <vilib>:"Space Constant.vi"() -> ("String"=w274:string)
        n132 = Concatenate Strings("Дата и время проведения:  " ("string"), w252, w274, w251) -> (w295:string)
        n133 = Concatenate Strings("Оператор:  " ("string"), w247) -> (w294:string)
        n134 = Concatenate Strings("Цель исследования:  " ("string"), w253) -> (w293:string)
        n135 = Concatenate Strings("Сплав:  " ("string"), w307) -> (w292:string)
        n136 = Concatenate Strings("Режим обработки:  " ("string"), w305) -> (w290:string)
        n137 = Concatenate Strings("Ванна:   " ("string"), w303) -> (w289:string)
        n138 = Number To Decimal String(number=w301) -> (decimal integer string=w300:string)  [unwired: 1 in]
        n139 = Array To Spreadsheet String(delimiter (Tab)="\t", array=w277, 3:"%3d" ("format string")) -> (spreadsheet string=w269:string)
        n140 = Concatenate Strings("Длительность процесса, мин:   " ("string"), w300) -> (w288:string)
        n141 = Concatenate Strings(w247, w248) -> (w246:string)
        n142 = Array To Spreadsheet String(delimiter (Tab)="\t", array=w298, 3:"%3d" ("format string")) -> (spreadsheet string=w296:string)
        n143 = call "File Dialog"("start path"=w267, "default name"=w246) -> ("selected path"=w262:path, "cancelled"=w263:bool, "error out"=w264:errorcluster)  [unwired: 10 in, 1 out]
        n144 = Concatenate Strings("Состав электролита:  " ("string"), "\r", w296) -> (w291:string)
        n145 = call "Read_Temp_Data_Log.vi"("DataLogPath"=w257) -> ("error out"=w254:errorcluster, "Data"=w255:string[][])  [unwired: 9 in]
        n146 = Build Array(w295, w294, w293, w292, w291, w290, w289, w288, w276, w276, w268, w269) -> (w287:string[])
        n147 = Strip Path(path=w262) -> (stripped path=w259:path, name=w261:string)
        n148 = Array To Spreadsheet String(delimiter (Tab)="\r", array=w287, 3:"%3d" ("format string")) -> (spreadsheet string=w265:string)
        n149 = Concatenate Strings(w261, "Oscill.txt" ("string")) -> (w258:string)
        n150 = case shown="False" w263 {
          tunnel: [w314 errorcluster {"status"=FALSE, "code"=0, "source"=""} ("error out")] -> w266
          tunnel: w262 -> [w313 _]
          tunnel: w265 -> [w312 _]
          tunnel: w264 -> [w311 _]
          frame False {
            w310 = u32 522252  # Зеленый
            n151 = Write to Text File(file (use dialog)=w313, text=w312, error in=w311) -> (refnum out=w315:refnum<file>, error out=w316:errorcluster)  [unwired: 1 in, 1 out]
            n152 = property on="ДАННЫЕ СОХРАНЕНЫ" class="Str"("Text.BGColor"=w310) -> ()  [unwired: 2 in, 2 out]
            n153 = Close File(refnum=w315, error in=w316) -> (error out=w314:errorcluster)  [unwired: 1 out]
          }
          frame True {
          }
        }
        n154 = Build Path(base path=w259, name or relative path=w258) -> (appended path=w256:path)
        n155 = call <vilib>:"Simple Error Handler.vi"("error in (no error)"=w254) -> ()  [unwired: 4 in, 5 out]
        n156 = call-poly <vilib>:"Write To Spreadsheet File.vi"("2D data"=w255, "file path (dialog if empty)"=w256) -> ()  [unwired: 6 in, 1 out]
        n157 = case shown="No Error" w266 {
          tunnel: w271 -> [w318 w320]
          tunnel: [w318 w319] -> w270
          frame No Error {
          }
          frame Error {
            w321 = T4[] [enum."Error_handler"] items=["Wait_for_event", "Initialize", "Save_ini", "Save_data", "Streaming_config", "Streaming_open", "Streaming_monitor", "Streaming_stop", "Vizualyze", "Form_data_fetch", "Process_analyze", "Start_data_loging", "Pause_data_loging", "Stop_data_loging", "Reset_data_colection", "Error_handler", "Stop", "Settings_dialog"] ("array")
            n158 = Build Array (concatenate)(w321, w320) -> (w319:T4[])
          }
        }
        n159 = Bundle By Name(cluster=w273, "Global_errors"=w266) -> (w272:T5)
      }
      frame "Streaming_config" {
        n160 = Unbundle By Name(w331) -> ("Streaming Refnum"=w346:refnum<vi>, "Options.Coeff_U"=w343:dbl, "Options.Offset_U"=w341:dbl, "Options.Coeff_I"=w340:dbl, "Options.Offset_I"=w337:dbl, "Modbus spy Refnum"=w329:refnum<vi>, "Options.VISA resource name"=w327:refnum<visa-resource-name>, "Options.Form_data_log_period"=w322:i32)
        n161 = call "Write_control_in_stream.vi"("Value"=w343, "Required_control_name"="Coeff_U", "reference"=w346) -> ("reference out"=w342:refnum<vi>)  [unwired: 8 in]
        n162 = call "Write_control_in_stream.vi"("Value"=w327, "Required_control_name"="VISA resource name", "reference"=w329) -> ("reference out"=w326:refnum<vi>)  [unwired: 8 in]
        n163 = call "Write_control_in_stream.vi"("Value"=w341, "Required_control_name"="Offset_U", "reference"=w342) -> ("reference out"=w339:refnum<vi>)  [unwired: 8 in]
        n164 = Close Reference(reference=w326) -> (error out=w324:errorcluster)  [unwired: 1 in]
        n165 = call "Write_control_in_stream.vi"("Value"=w340, "Required_control_name"="Coeff_I", "reference"=w339) -> ("reference out"=w336:refnum<vi>)  [unwired: 8 in]
        n166 = call "Write_control_in_stream.vi"("Value"=w337, "Required_control_name"="Offset_I", "reference"=w336) -> ("reference out"=w334:refnum<vi>)  [unwired: 8 in]
        n167 = property on="FormCharts" class="WFChart (strict)"("XScale.Multiplier"=w322) -> ()  [unwired: 2 in, 2 out]
        n168 = Close Reference(reference=w334) -> (error out=w325:errorcluster)  [unwired: 1 in]
        n169 = Merge Errors(w325, w324) -> (w323:errorcluster)
        n170 = case shown="No Error" w323 {
          tunnel: w333 -> [w347 w350]
          tunnel: [w347 w349] -> w332
          frame No Error {
          }
          frame Error {
            w348 = T4[] [enum."Error_handler"] items=["Wait_for_event", "Initialize", "Save_ini", "Save_data", "Streaming_config", "Streaming_open", "Streaming_monitor", "Streaming_stop", "Vizualyze", "Form_data_fetch", "Process_analyze", "Start_data_loging", "Pause_data_loging", "Stop_data_loging", "Reset_data_colection", "Error_handler", "Stop", "Settings_dialog"] ("array")
            n171 = Build Array (concatenate)(w348, w350) -> (w349:T4[])
          }
        }
        n172 = Bundle By Name(cluster=w331, "Global_errors"=w323) -> (w330:T5)
      }
      frame "Streaming_open" {
        n173 = Unbundle By Name(w361) -> ("Streaming Refnum"=w357:refnum<vi>, "Modbus spy Refnum"=w351:refnum<vi>)
        n174 = invoke class="VI" method="Run VI"(reference=w357, "Wait until done"=FALSE ("Wait Until Done")) -> (reference out=w358:refnum<vi>, error out=w359:errorcluster)  [unwired: 3 in, 3 out]
        n175 = invoke class="VI" method="Run VI"(reference=w351, "Wait until done"=FALSE ("Wait Until Done")) -> (reference out=w354:refnum<vi>, error out=w353:errorcluster)  [unwired: 3 in, 3 out]
        n176 = Close Reference(reference=w358, error in (no error)=w359) -> (error out=w356:errorcluster)
        n177 = Close Reference(reference=w354, error in (no error)=w353) -> (error out=w355:errorcluster)
        n178 = call <vilib>:"Clear Errors.vi"("error in (no error)"=w356) -> ()  [unwired: 6 in, 1 out]
        n179 = call <vilib>:"Clear Errors.vi"("error in (no error)"=w355) -> ()  [unwired: 6 in, 1 out]
        n180 = Bundle By Name(cluster=w361, "Streaming_enable"=TRUE) -> (w363:T5)
      }
      frame "Streaming_monitor" {
        (unwired) waveform(dbl) {"t0"=timestamp(0 s since 1904-01-01), "dt"=1.0, "Y"=[]} ("output waveform")
        w391 = dbl[] []
        w376 = "error out" ("Required_indicatorl_name")
        n181 = Unbundle By Name(w403) -> ("Streaming Refnum"=w402:refnum<vi>, "Modbus spy Refnum"=w387:refnum<vi>, "Options.ADC_frequency"=w369:dbl)
        n182 = Reciprocal(x=w369) -> (1/x=w366:dbl)
        n183 = call "Read_indicator_in_stream.vi"("Required_indicatorl_name"="Напряжение", "reference"=w402) -> ("error out"=w383:errorcluster, "Value"=w392:variant, "reference out"=w401:refnum<vi>)  [unwired: 7 in]
        n184 = call "Read_indicator_in_stream.vi"("Required_indicatorl_name"="MBA data", "reference"=w387) -> ("error out"=w378:errorcluster, "Value"=w385:variant, "reference out"=w377:refnum<vi>)  [unwired: 7 in]
        n185 = Variant To Data(error in=w383, type=w391, Variant=w392) -> (data=w371:dbl[], error out=w382:errorcluster)
        n186 = call "Read_indicator_in_stream.vi"("error in (no error)"=w382, "Required_indicatorl_name"="Ток", "reference"=w401) -> ("error out"=w381:errorcluster, "Value"=w397:variant, "reference out"=w400:refnum<vi>)  [unwired: 6 in]
        n187 = Variant To Data(error in=w378, type=T9 {"MBA_ch 1"=0.0, "MBA_ch 2"=0.0, "MBA_ch 3"=0.0, "MBA_ch 4"=0.0, "MBA_ch 5"=0.0, "MBA_ch 6"=0.0, "MBA_ch 7"=0.0, "MBA_ch 8"=0.0} ("MBA data"), Variant=w385) -> (data=w386:T9, error out=w374:errorcluster)
        n188 = disable-structure shown="Enabled" {
          disable-tunnel: w377 -> [w415 w417]
          disable-tunnel: w376 -> [w414 _]
          disable-tunnel: w374 -> [w409 _]
          disable-tunnel: [w408 w416] -> w373
          disable-tunnel: [w407 w416] -> w372
          frame Disabled {
            n189 = call "Read_indicator_in_stream.vi"("Required_indicatorl_name"=w414, "reference"=w415) -> ("error out"=w413:errorcluster, "Value"=w410:variant, "reference out"=w411:refnum<vi>)  [unwired: 7 in]
            n190 = Close Reference(reference=w411, error in (no error)=w413) -> (error out=w412:errorcluster)
            n191 = Variant To Data(error in=w412, type=w409, Variant=w410) -> (data=w408:errorcluster, error out=w407:errorcluster)
          }
          frame Enabled {
            n192 = Close Reference(reference=w417) -> (error out=w416:errorcluster)  [unwired: 1 in]
          }
        }
        n193 = Variant To Data(error in=w381, type=w391, Variant=w397) -> (data=w370:dbl[], error out=w380:errorcluster)
        n194 = call "Read_indicator_in_stream.vi"("error in (no error)"=w380, "Required_indicatorl_name"=w376, "reference"=w400) -> ("error out"=w379:errorcluster, "Value"=w396:variant, "reference out"=w395:refnum<vi>)  [unwired: 6 in]
        n195 = Bundle By Name("dt"=w366) -> (w365:waveform(dbl))  [unwired: 1 in]
        n196 = Close Reference(reference=w395, error in (no error)=w379) -> (error out=w375:errorcluster)
        n197 = Bundle By Name(cluster=w365, "Y"=w371) -> (w368:waveform(dbl))
        n198 = Bundle By Name(cluster=w365, "Y"=w370) -> (w367:waveform(dbl))
        n199 = Variant To Data(error in=w375, type=w375, Variant=w396) -> (data=w393:errorcluster, error out=w394:errorcluster)
        n200 = Merge Errors(w393, w394, w374, w373, w372) -> (w389:errorcluster)
        n201 = Not(x=w389) -> (.not. x?=w390:bool)
        n202 = case shown="No Error" w389 {
          tunnel: w406 -> [w418 w421]
          tunnel: [w418 w420] -> w405
          frame No Error {
          }
          frame Error {
            w419 = T4[] [enum."Error_handler"] items=["Wait_for_event", "Initialize", "Save_ini", "Save_data", "Streaming_config", "Streaming_open", "Streaming_monitor", "Streaming_stop", "Vizualyze", "Form_data_fetch", "Process_analyze", "Start_data_loging", "Pause_data_loging", "Stop_data_loging", "Reset_data_colection", "Error_handler", "Stop", "Settings_dialog"] ("array")
            n203 = Build Array (concatenate)(w421, w419) -> (w420:T4[])
          }
        }
        n204 = Bundle By Name(cluster=w403, "Voltege waveform"=w368, "Current waveform"=w367, "Global_errors"=w389, "Streaming_enable"=w390, "MBA data"=w386) -> (w404:T5)
      }
      frame "Streaming_stop" {
        w426 = TRUE
        w427 = "Стоп" ("Required_control_name")
        w434 = FALSE ("Streaming_enable")
        n205 = Unbundle By Name(w433) -> ("Streaming Refnum"=w432:refnum<vi>, "Modbus spy Refnum"=w425:refnum<vi>)
        n206 = call "Write_control_in_stream.vi"("Value"=w426, "Required_control_name"=w427, "reference"=w432) -> ("reference out"=w431:refnum<vi>)  [unwired: 8 in]
        n207 = call "Write_control_in_stream.vi"("Value"=w426, "Required_control_name"=w427, "reference"=w425) -> ("reference out"=w428:refnum<vi>)  [unwired: 8 in]
        n208 = Close Reference(reference=w428) -> (error out=w423:errorcluster)  [unwired: 1 in]
        n209 = Close Reference(reference=w431) -> (error out=w424:errorcluster)  [unwired: 1 in]
        n210 = Merge Errors(w424, w423) -> (w422:errorcluster)
        n211 = case shown="Error" w422 {
          tunnel: w430 -> [w436 w438]
          tunnel: [w436 w437] -> w429
          frame No Error {
          }
          frame Error {
            w439 = T4[] [enum."Error_handler"] items=["Wait_for_event", "Initialize", "Save_ini", "Save_data", "Streaming_config", "Streaming_open", "Streaming_monitor", "Streaming_stop", "Vizualyze", "Form_data_fetch", "Process_analyze", "Start_data_loging", "Pause_data_loging", "Stop_data_loging", "Reset_data_colection", "Error_handler", "Stop", "Settings_dialog"] ("array")
            n212 = Build Array (concatenate)(w439, w438) -> (w437:T4[])
          }
        }
        n213 = Bundle By Name(cluster=w433, "Streaming_enable"=w434, "Data_write_enable"=w434, "Global_errors"=w422) -> (w435:T5)
      }
      frame "Vizualyze" {
        # "Амплитудное значение напряжения"
        n214 = Unbundle By Name(w467) -> ("Process conditions.Bath volume"=w454:string, "MBA data"=w455:T9, "Voltege waveform"=w440:waveform(dbl), "Current waveform"=w442:waveform(dbl), "Data_write_enable"=w465:bool, "Options.startup_threshold"=w466:dbl)
        "Bath type" <- w454
        n215 = Unbundle By Name(w455) -> ("MBA_ch 3"=w451:dbl, "MBA_ch 7"=w450:dbl, "MBA_ch 6"=w447:dbl)
        n216 = Bundle("Voltege waveform"=w440, "Current waveform"=w442) -> (→"Mixed Signal Graph":T2)  [unwired: 1 in]
        n217 = Greater?(x=w451, y=10.0) -> (0:→"Ventilation flow":bool)
        n218 = Greater?(x=w450, y=80.0) -> (0:→"Bubbling flow":bool)
        n219 = Multiply(x=w447, y=1.0) -> (x*y=→"Cooler flow":dbl)
        n220 = Unbundle By Name(w440) -> ("Y"=w457:dbl[])
        n221 = Array Max & Min(array=w457) -> (max value=w456:dbl)  [unwired: 3 out]
        n222 = Not(x=w465) -> (.not. x?=w463:bool)
        n223 = Greater?(x=w456, y=w466) -> (0:w464:bool)
        n224 = Compound Arithmetic op=AND(w464, w463, "Отложенный запуск") -> (w461:bool)
        n225 = case shown="True" w461 {
          tunnel: [w476 w477] -> w458
          frame False {
            w476 = T4[] [] items=["Wait_for_event", "Initialize", "Save_ini", "Save_data", "Streaming_config", "Streaming_open", "Streaming_monitor", "Streaming_stop", "Vizualyze", "Form_data_fetch", "Process_analyze", "Start_data_loging", "Pause_data_loging", "Stop_data_loging", "Reset_data_colection", "Error_handler", "Stop", "Settings_dialog"] ("array")
          }
          frame True {
            w477 = T4[] [enum."Start_data_loging"] items=["Wait_for_event", "Initialize", "Save_ini", "Save_data", "Streaming_config", "Streaming_open", "Streaming_monitor", "Streaming_stop", "Vizualyze", "Form_data_fetch", "Process_analyze", "Start_data_loging", "Pause_data_loging", "Stop_data_loging", "Reset_data_colection", "Error_handler", "Stop", "Settings_dialog"] ("array")
            n226 = local write "Отложенный запуск"(FALSE ("Отложенный запуск")) -> ()
          }
        }
        n227 = case shown="\"2000 л\"" w454 {
          tunnel: w455 -> [w469 w471 w473 w475]
          tunnel: [w468 w470 w472 w474] -> w444
          frame "30 л", Default {
            n228 = Unbundle By Name(w469) -> ("MBA_ch 4"=w468:dbl)
          }
          frame "80 л" {
            n229 = Unbundle By Name(w471) -> ("MBA_ch 1"=w470:dbl)
          }
          frame "800 л" {
            n230 = Unbundle By Name(w473) -> ("MBA_ch 5"=w472:dbl)
          }
          frame "2000 л" {
            n231 = Unbundle By Name(w475) -> ("MBA_ch 8"=w474:dbl)
          }
        }
        "Electrolyte temperature" <- w444
        n232 = call "Termometr_color.vi"("Temperature"=w444) -> ("Scale color"=w443:u32)  [unwired: 8 in]
        n233 = property on="Electrolyte temperature" class="Slide (strict)"("Fill Color"=w443) -> ()  [unwired: 2 in, 2 out]
        n234 = Build Array (concatenate)(w460, w458) -> (w459:T4[])
      }
      frame "Form_data_fetch" {
        n235 = Unbundle By Name(w514) -> ("Data log path"=w516:path, "Process_time"=w523:u32, "Voltege waveform"=w480:waveform(dbl), "Current waveform"=w479:waveform(dbl))
        n236 = Divide(x=w523, y=u32 60000) -> (x/y=w522:dbl)
        n237 = call "A-K_meas.vi"("Input wave"=w480) -> ("Katod_dbl"=w496:T14, "Katod_str"=w512:T15, "Anod_dbl"=w497:T16, "Anod_str"=w513:T17)  [unwired: 7 in]
        n238 = call "A-K_meas.vi"("Input wave"=w479) -> ("Katod_dbl"=w494:T14, "Katod_str"=w510:T15, "Anod_dbl"=w495:T16, "Anod_str"=w511:T17)  [unwired: 7 in]
        n239 = local read "Electrolyte temperature"() -> (w519:dbl)
        n240 = Number To Fractional String(number=w522, precision (6)=i16 1 ("width (-)")) -> (F-format string=w520:string)  [unwired: 2 in]
        n241 = Concatenate Strings(w520, " мин" ("string")) -> (w515:string)
        n242 = Number To Fractional String(number=w519, precision (6)=i16 1 ("width (-)")) -> (F-format string=w518:string)  [unwired: 2 in]
        n243 = Unbundle By Name(w512) -> ("Katod_amp"=w499:string, "Katod_rms"=w503:string, "Katod_mean"=w507:string)
        n244 = Unbundle By Name(w510) -> ("Katod_amp"=w498:string, "Katod_rms"=w502:string, "Katod_mean"=w506:string)
        n245 = Unbundle By Name(w513) -> ("Anod_amp"=w501:string, "Anod_rms"=w505:string, "Anod_mean"=w509:string)
        n246 = Unbundle By Name(w511) -> ("Anod_amp"=w500:string, "Anod_rms"=w504:string, "Anod_mean"=w508:string)
        n247 = Unbundle(w497) -> ("Anod_amp"=w493:dbl, "Anod_rms"=w492:dbl, "Anod_mean"=w491:dbl)
        n248 = Unbundle(w496) -> ("Katod_amp"=w490:dbl, "Katod_rms"=w489:dbl, "Katod_mean"=w488:dbl)
        n249 = Unbundle(w495) -> ("Anod_amp"=w487:dbl, "Anod_rms"=w486:dbl, "Anod_mean"=w485:dbl)
        n250 = Unbundle(w494) -> ("Katod_amp"=w484:dbl, "Katod_rms"=w483:dbl, "Katod_mean"=w482:dbl)
        n251 = disable-structure shown="Enabled" {
          disable-tunnel: w516 -> [w534 _]
          disable-tunnel: w515 -> [w533 _]
          disable-tunnel: w480 -> [w531 _]
          disable-tunnel: w479 -> [w530 _]
          frame Enabled {
            n252 = call "Write_Temp_Data_Log.vi"("Process_time"=w533, "Current (A)"=w530, "Voltage (V)"=w531, "datalog path (use dialog)"=w534) -> ("error out"=w532:errorcluster)  [unwired: 7 in]
            n253 = call <vilib>:"Simple Error Handler.vi"("error in (no error)"=w532) -> ()  [unwired: 4 in, 5 out]
          }
          frame Disabled {
          }
        }
        n254 = Bundle("Anod_amp"=w493, "Anod_rms"=w492, "Anod_mean"=w491, "Katod_amp"=w490, "Katod_rms"=w489, "Katod_mean"=w488, "Anod_amp"=w487, "Anod_rms"=w486, "Anod_mean"=w485, "Katod_amp"=w484, "Katod_rms"=w483, "Katod_mean"=w482) -> (→"FormCharts":T3)  [unwired: 1 in]
        n255 = local read "Process Electrical Parameters"() -> (w528:string[][])
        n256 = Build Array(w515, w509, w508, w507, w506, w505, w504, w503, w502, w501, w500, w499, w498, w518) -> (w527:string[])
        n257 = Build Array (concatenate)(w528, w527) -> (→"Process Electrical Parameters":string[][])
      }
      frame "Process_analyze" {
        w562 = 5  # i
        # "Амплитудное значение напряжения"
        # "Усреднение значения на основе i измерений"
        n258 = Unbundle By Name(w550) -> ("Data_write_enable"=w536:bool, "Voltege waveform"=w544:waveform(dbl))
        n259 = Unbundle By Name(w544) -> ("Y"=w546:dbl[])
        n260 = Array Max & Min(array=w546) -> (max value=w545:dbl)  [unwired: 3 out]
        n261 = local read "Max_voltage"() -> (w540:dbl)
        n262 = feedback #4(dbl[] []) -> (w561:dbl[])
        n263 = Build Array (concatenate)(w561, w545) -> (w563:dbl[])
        n264 = Delete From Array(array=w563, length=w562) -> (deleted portion=w559:dbl[])  [unwired: 1 in, 1 out]
        n265 = feedback-in #4(w559) -> ()
        n266 = call-poly <vilib>:"Mean.vi"("X"=w559) -> ("mean"=w541:dbl)  [unwired: 1 out]
        n267 = Multiply(x=w540, y=0.9) -> (x*y=w557:dbl)
        n268 = Less?(x=w541, y=w557) -> (x < y?=w556:bool)
        n269 = local read "Пауза"() -> (w537:bool)
        n270 = Greater?(x=w541, y=w540) -> (0:w542:bool)
        n271 = property on="УГАСАНИЕ" class="Str"() -> ("Text.BGColor"=w538:u32)  [unwired: 2 in, 2 out]
        n272 = Select(t=w541, s=w542, f=w540) -> (s? t:f=w539:dbl)
        n273 = Or(x=w537, y=w536) -> (x .or. y?=w535:bool)
        n274 = case shown="True" w535 {
          tunnel: w556 -> [_ w578]
          tunnel: [w564 w577] -> w555
          tunnel: w541 -> [_ w576]
          tunnel: [w567 w575] -> w554
          tunnel: [w567 w574] -> w553
          tunnel: [w567 w573] -> w552
          tunnel: [w567 w572] -> w551
          tunnel: w549 -> [w566 w571]
          tunnel: [w566 w570] -> w548
          tunnel: "StopUgasanie" -> [_ w569]
          tunnel: [0.0 w568] -> w543
          tunnel: w539 -> [_ w568]
          tunnel: w538 -> [w564 _]
          frame False {
            w567 = 3158064  # Темно-серый
          }
          frame True {
            n275 = case shown="True" w578 {
              tunnel: [w593 w601] -> w577
              tunnel: [w592 w600] -> w572
              tunnel: [w591 w600] -> w573
              tunnel: [w590 w600] -> w574
              tunnel: [w589 w600] -> w575
              tunnel: w576 -> [w583 _]
              tunnel: w571 -> [w579 w599]
              tunnel: [w579 w598] -> w570
              tunnel: w569 -> [_ w597]
              frame False {
                w581 = 400.0 ("upper limit")
                w580 = 600.0 ("upper limit")
                w584 = 800.0 ("upper limit")
                w588 = 522252  # Зеленый
                w593 = 3158064  # Темно-серый
                # "Развитие МДР"
                n276 = Greater?(x=w583, y=w584) -> (0:w585:bool)
                n277 = Less?(x=w583, y=w581) -> (x < y?=w582:bool)
                n278 = In Range and Coerce(upper limit=w584, x=w583, lower limit=w580) -> (In Range?=w587:bool)  [unwired: 1 out]
                n279 = In Range and Coerce(upper limit=w580, x=w583, lower limit=w581) -> (In Range?=w586:bool)  [unwired: 1 out]
                n280 = Select(t=w588, s=w585, f=w593) -> (s? t:f=w592:i32)
                n281 = Select(t=w588, s=w587, f=w593) -> (s? t:f=w591:i32)
                n282 = Select(t=w588, s=w586, f=w593) -> (s? t:f=w590:i32)
                n283 = Select(t=w588, s=w582, f=w593) -> (s? t:f=w589:i32)
              }
              frame True {
                w595 = T4[] [] items=["Wait_for_event", "Initialize", "Save_ini", "Save_data", "Streaming_config", "Streaming_open", "Streaming_monitor", "Streaming_stop", "Vizualyze", "Form_data_fetch", "Process_analyze", "Start_data_loging", "Pause_data_loging", "Stop_data_loging", "Reset_data_colection", "Error_handler", "Stop", "Settings_dialog"] ("array")
                w596 = T4[] [enum."Stop_data_loging"] items=["Wait_for_event", "Initialize", "Save_ini", "Save_data", "Streaming_config", "Streaming_open", "Streaming_monitor", "Streaming_stop", "Vizualyze", "Form_data_fetch", "Process_analyze", "Start_data_loging", "Pause_data_loging", "Stop_data_loging", "Reset_data_colection", "Error_handler", "Stop", "Settings_dialog"] ("array")
                w600 = 3158064  # Темно-серый
                w601 = 16254993  # Красный
                # "Угасание"
                n284 = Select(t=w596, s=w597, f=w595) -> (s? t:f=w594:T4[])
                n285 = Build Array (concatenate)(w599, w594) -> (w598:T4[])
              }
            }
          }
        }
        "Max_voltage" <- w543
        n286 = property on="ДР" class="Str"("Text.BGColor"=w551) -> ()  [unwired: 2 in, 2 out]
        n287 = property on="МДР" class="Str"("Text.BGColor"=w552) -> ()  [unwired: 2 in, 2 out]
        n288 = property on="ИР" class="Str"("Text.BGColor"=w553) -> ()  [unwired: 2 in, 2 out]
        n289 = property on="ГАЛЬВ.ЛЮМ." class="Str"("Text.BGColor"=w554) -> ()  [unwired: 2 in, 2 out]
        n290 = property on="УГАСАНИЕ" class="Str"("Text.BGColor"=w555) -> ()  [unwired: 2 in, 2 out]
      }
      frame "Start_data_loging" {
        n291 = in-place {
          w605 = u32 3158064 ("Темно-серый")
          w609 = T12."Enabled" ("Disabled")
          n292 = in-place-cluster #5(w603) -> ("Streaming_enable"=w608:bool)  [unwired: 2 out]
          n293 = Select(t=u32 522252 ("Зеленый"), s=w608, f=w605) -> (s? t:f=w606:u32)
          n294 = property on="СБОР" class="Str"("Text.BGColor"=w606) -> ()  [unwired: 2 in, 2 out]
          n295 = property on="ДАННЫЕ СОХРАНЕНЫ" class="Str"("Text.BGColor"=w605) -> ()  [unwired: 2 in, 2 out]
          n296 = property on="Пауза" class="Bool (strict)"("DisabledEnum"=w609) -> ()  [unwired: 2 in, 2 out]
          n297 = property on="СТОП" class="Bool (strict)"("DisabledEnum"=w609) -> ()  [unwired: 2 in, 2 out]
          n298 = Tick Count (ms)() -> (millisecond timer value=w610:u32)
          n299 = in-place-cluster #5("Streaming_enable"=w608, "Data_write_enable"=w608, "startup_time"=w610) -> (w602:T5)
        }
      }
      frame "Pause_data_loging" {
      }
      frame "Stop_data_loging" {
        w613 = T12."Disabled" ("Disabled")
        n300 = property on="Пауза" class="Bool (strict)"("DisabledEnum"=w613) -> ()  [unwired: 2 in, 2 out]
        n301 = property on="СТОП" class="Bool (strict)"("DisabledEnum"=w613) -> ()  [unwired: 2 in, 2 out]
      }
      frame "Reset_data_colection" {
        w617 = 3158064  # Темно-серый
        n302 = Unbundle By Name(w619) -> ("Data log path"=w618:path)
        n303 = property on="FormCharts" class="WFChart (strict)"("History Data"=T10 []) -> ()  [unwired: 2 in, 2 out]
        n304 = local write "Process Electrical Parameters"(string[][] [] ("Process Electrical Parameters")) -> ()
        n305 = Open/Create/Replace Datalog(5:cluster{string, "empty array":sgl[]} {"", "empty array"=[]}, 10:T11."replace" ("operation (0:open)"), 11:w618) -> (0:w621:errorcluster, 3:w620:refnum<k1>)  [unwired: 1 in, 3 out]
        n306 = Close File(refnum=w620, error in=w621) -> ()  [unwired: 2 out]
        n307 = local write "Max_voltage"(0.0 ("Max_voltage")) -> ()
        n308 = property on="ДАННЫЕ СОХРАНЕНЫ" class="Str"("Text.BGColor"=w617) -> ()  [unwired: 2 in, 2 out]
      }
      frame "Error_handler" {
        n309 = in-place {
          in-place-border: w628 -> [w637]
          in-place-border: [w636] -> w627
          w635 = T4[] [enum."Streaming_stop", enum."Streaming_config", enum."Streaming_open"] items=["Wait_for_event", "Initialize", "Save_ini", "Save_data", "Streaming_config", "Streaming_open", "Streaming_monitor", "Streaming_stop", "Vizualyze", "Form_data_fetch", "Process_analyze", "Start_data_loging", "Pause_data_loging", "Stop_data_loging", "Reset_data_colection", "Error_handler", "Stop", "Settings_dialog"] ("array")
          n310 = in-place-cluster #6(w630) -> ("Global_errors"=w631:errorcluster)
          n311 = feedback-in #7(w631) -> ()
          n312 = feedback #7(errorcluster {"status"=FALSE, "code"=0, "source"=""} ("Global_errors")) -> (w633:errorcluster)
          n313 = Equal?(x=w631, y=w633) -> (x = y?=w632:bool)
          n314 = case shown="False" w632 {
            tunnel: w631 -> [w640 _]
            frame False {
              w639 = T18 3 items=["no dialog", "OK message", "continue or stop message", "OK message + warnings", "continue/stop + warnings"] ("type of dialog (OK msg:1)")
              n315 = call <vilib>:"General Error Handler.vi"("type of dialog (OK msg:1)"=w639, "error in (no error)"=w640) -> ()  [unwired: 9 in, 5 out]
            }
            frame True {
            }
          }
          n316 = Build Array (concatenate)(w637, w635) -> (w636:T4[])
          n317 = in-place-cluster #6("Global_errors"=errorcluster {"status"=FALSE, "code"=0, "source"=""}) -> (w629:T5)
        }
      }
      frame "Stop" {
      }
      frame "Settings_dialog" {
        n318 = Unbundle By Name(w647) -> ("Ini_file_path"=w650:path)
        n319 = call "Read_INI.vi"("App_directory"=w650) -> ("Options"=w649:T6)  [unwired: 8 in, 2 out]
        n320 = call "Settings_dialog.vi"("Options"=w649) -> ("Canceled"=w648:bool, "Options_out"=w645:T6)  [unwired: 9 in]
        n321 = case shown="False" w648 {
          tunnel: w647 -> [w653 w658]
          tunnel: w646 -> [w656 w657]
          tunnel: w645 -> [w652 _]
          tunnel: [w654 w657] -> w644
          tunnel: [w651 w658] -> w643
          frame False {
            w655 = T4[] [enum."Save_ini", enum."Streaming_stop", enum."Streaming_config", enum."Streaming_open"] items=["Wait_for_event", "Initialize", "Save_ini", "Save_data", "Streaming_config", "Streaming_open", "Streaming_monitor", "Streaming_stop", "Vizualyze", "Form_data_fetch", "Process_analyze", "Start_data_loging", "Pause_data_loging", "Stop_data_loging", "Reset_data_colection", "Error_handler", "Stop", "Settings_dialog"] ("array")
            n322 = Bundle By Name(cluster=w653, "Options"=w652) -> (w651:T5)
            n323 = Build Array (concatenate)(w656, w655) -> (w654:T4[])
          }
          frame True {
          }
        }
      }
    }
    n324 = Equal?(x=w8, y=main_states."Stop") -> (x = y?=w23:bool)
    n325 = property on="current_state" class="Enum (strict)"() -> ("RingText.Text"=w20:string)  [unwired: 2 in, 2 out]
    n326 = feedback #8("") -> (w11:string)
    n327 = Concatenate Strings(w20, "\r", w11) -> (w21:string)
    n328 = String Subset(string=w21, length (rest)=1000 ("length (rest)")) -> (substring=w17:string)  [unwired: 1 in]
    "states_history" <- w17
    n329 = feedback-in #8(w17) -> ()
  }
  n330 = Unbundle By Name(w5) -> ("shutdown?"=w1:bool)
  n331 = property class="App"() -> (reference out=w4:refnum<vi>, error out=w3:errorcluster, "App.Kind"=w2:T13)  [unwired: 2 in]
  n332 = Close Reference(reference=w4, error in (no error)=w3) -> ()  [unwired: 1 out]
  n333 = case shown="\"Run Time System\"" w2 {
    tunnel: w1 -> [_ w659]
    frame "Development System", Default {
    }
    frame "Run Time System" {
      n334 = stacked-sequence {
        tunnel: w659 -> [w660 _]
        frame #0 {
          n335 = case shown="True" w660 {
            frame False {
            }
            frame True {
              n336 = call <vilib>:"System Exec.vi"("command line"="Shutdown /s /t 0") -> ()  [unwired: 7 in, 4 out]
            }
          }
        }
        frame #1 {
          n337 = Quit LabVIEW(quit? (T)=TRUE) -> ()
        }
      }
    }
  }
